vi "test.vi"() -> ()   [LabVIEW 2010]
uses:
  <vilib>/Utility/miscctls.llb/LVPositionTypeDef.ctl
  <vilib>/Utility/miscctls.llb/LVBoundsTypeDef.ctl
  <vilib>/Utility/miscctls.llb/LVFontTypeDef.ctl
  Classes/Control/Control.lvclass
  Classes/Control/init/init control_string.vi
  Classes/Control/init/init control_path.vi
panel:
  in  "ignore caption & label? (T)":bool=TRUE
  in  "Font":T1={"Font Name"="Arial", "Size"=14, "Bold"=FALSE, "Italic"=FALSE, "Underline"=FALSE, "Strikeout"=FALSE, "Color"=0}
  out "Array":T4(array[cluster])
  out "error out":errorcluster
  in  "Path":path=path "C:/"
  in  "String":string="string"
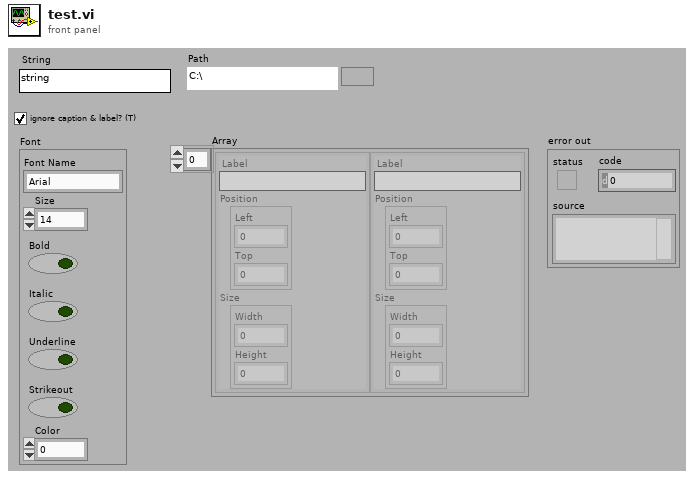
[diagram p1: front panel]
types:
  T1 = typedef "LVFontTypeDef.ctl" = cluster{"Font Name":string, "Size":u16, "Bold":bool, "Italic":bool, "Underline":bool, "Strikeout":bool, "Color":u32}
  T2 = typedef "LVPositionTypeDef.ctl" = cluster{"Left":i32, "Top":i32}
  T3 = typedef "LVBoundsTypeDef.ctl" = cluster{"Width":u32, "Height":u32}
  T4 = cluster{"Label":string, "Position":T2, "Size":T3}[]
  T5 = cluster{"Label":string, "Position":T2, "Size":T3}
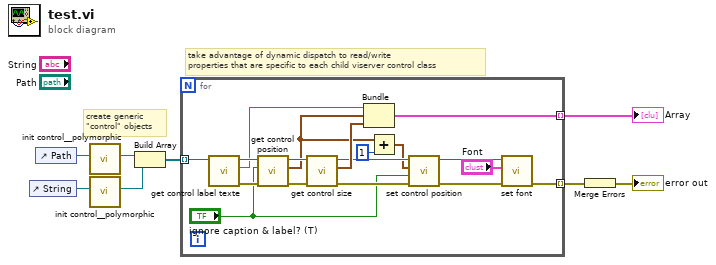
[diagram p0: block diagram]
diagram:
  # "take advantage of dynamic dispatch to read/write\nproperties that are specific to each child viserver control class"
  # "create generic\n\"control\" objects"
  n1 = control-ref of="String"() -> (w1:refnum<vi>)
  n2 = control-ref of="Path"() -> (w2:refnum<vi>)
  n3 = call-poly "init control__polymorphic.vi"("Path Refnum"=w2) -> ("Control out"=w3:refnum<class "Control.lvclass">)  [unwired: 10 in]
  n4 = call-poly "init control__polymorphic.vi"("Str Refnum"=w1) -> ("Control out"=w4:refnum<class "Control.lvclass">)  [unwired: 10 in]
  n5 = Build Array(w3, w4) -> (w8:refnum<class "Control.lvclass">[])
  n6 = for {
    tunnel: w8 -> [w26] mode=indexing
    tunnel: [w18] -> w7 mode=indexing
    tunnel: [w19] -> w5 mode=indexing
    n7 = call-dynamic "get control label texte.vi"("Control in"=w26) -> ("error out"=w22:errorcluster, "Label"=w21:string, "Control out"=w25:refnum<class "Control.lvclass">)  [unwired: 8 in]
    n8 = call-dynamic "get control position.vi"("error in (no error)"=w22, "ignore caption & label? (T)"="ignore caption & label? (T)", "Control in"=w25) -> ("error out"=w23:errorcluster, "Position"=w11:T2, "Control out"=w24:refnum<class "Control.lvclass">)  [unwired: 6 in]
    n9 = call-dynamic "get control size.vi"("error in (no error)"=w23, "Control in"=w24) -> ("error out"=w15:errorcluster, "Size"=w20:T3, "Control out"=w16:refnum<class "Control.lvclass">)  [unwired: 7 in]
    n10 = Bundle("Label"=w21, "Position"=w11, "Size"=w20) -> (w19:T5)  [unwired: 1 in]
    n11 = Add(x=w11, y=1) -> (x+y=w10:T2)
    n12 = call-dynamic "set control position.vi"("error in (no error)"=w15, "ignore caption & label? (T)"="ignore caption & label? (T)", "Position"=w10, "Control in"=w16) -> ("error out"=w14:errorcluster, "Control out"=w13:refnum<class "Control.lvclass">)  [unwired: 6 in]
    n13 = call-dynamic "set font.vi"("error in (no error)"=w14, "Font"="Font", "Control in"=w13) -> ("error out"=w18:errorcluster)  [unwired: 7 in, 1 out]
  }
  "Array" <- w5
  n14 = Merge Errors(w7) -> (→"error out":errorcluster)
